vi "Get Unix Time.vi"() -> (3 "Unix Timestamp":dbl)   [LabVIEW 2016]
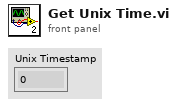
[diagram p1: front panel]
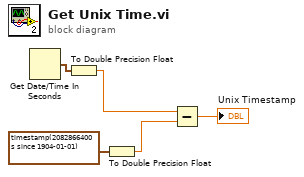
[diagram p0: block diagram]
diagram:
  n1 = Get Date/Time In Seconds() -> (seconds since 1Jan1904=w5:timestamp)
  n2 = To Double Precision Float(number=w5) -> (double precision float=w3:dbl)
  n3 = To Double Precision Float(number=timestamp(2082866400 s since 1904-01-01) ("current time")) -> (double precision float=w2:dbl)
  n4 = Subtract(x=w3, y=w2) -> (x-y=→"Unix Timestamp":dbl)
